vi "4.6.3.vi"() -> ()   [LabVIEW 2017]
panel:
  in  "停止":bool
  out "结果":dbl
  in  "b":dbl
  in  "a":dbl
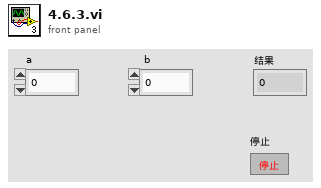
[diagram p1: front panel]
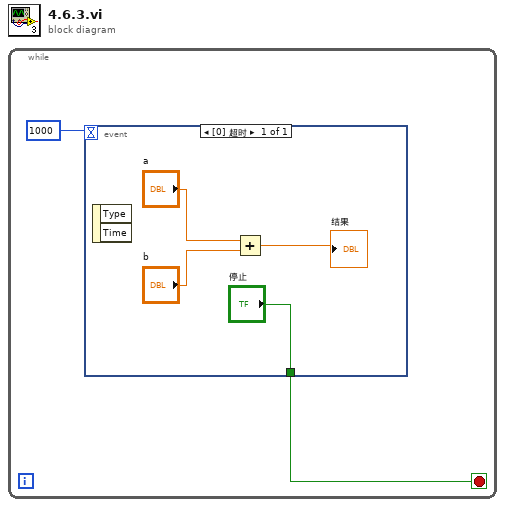
[diagram p0: block diagram]
diagram:
  n1 = while {
    stop <- w1 stop-if-true
    n2 = event shown="[0] 超时" {
      selector: _ -> [_]
      dyn-events: _ -> [_]
      timeout: 1000 -> [_]
      tunnel: ["停止"] -> w1
      event Timeout {
        n3 = event-data() -> ()  [unwired: 1 in, 2 out]
        n4 = Add(x="a", y="b") -> (x+y=→"结果":dbl)
      }
    }
  }
